vi "Generation of code word using msg and generator matrix(SubVI).vi"(1 "G in":dbl[][](array[numeric]), 2 "messages in":i16[][](array[numeric]), 3 "k":i32, 4 "n":i32) -> (0 "CODEWORDS":i32[][](array[numeric]))   [LabVIEW 2014]
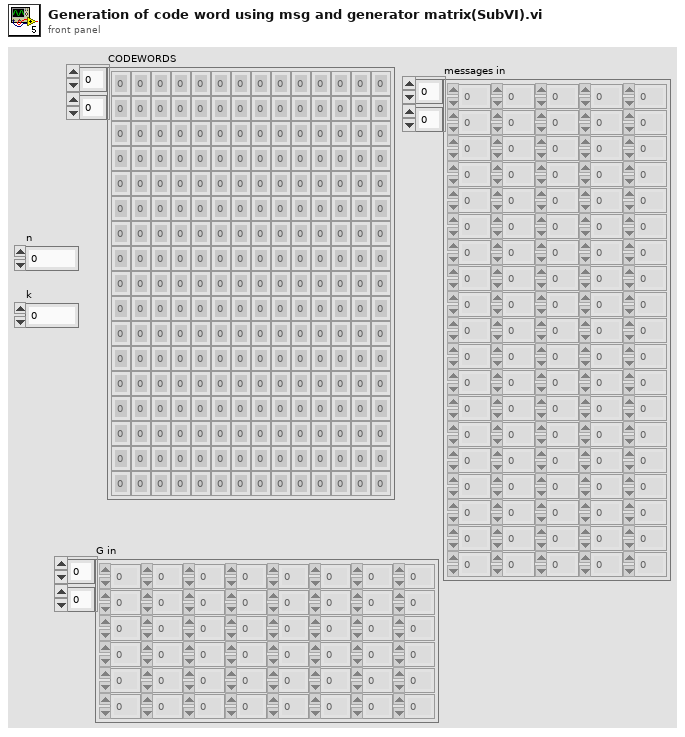
[diagram p1: front panel]
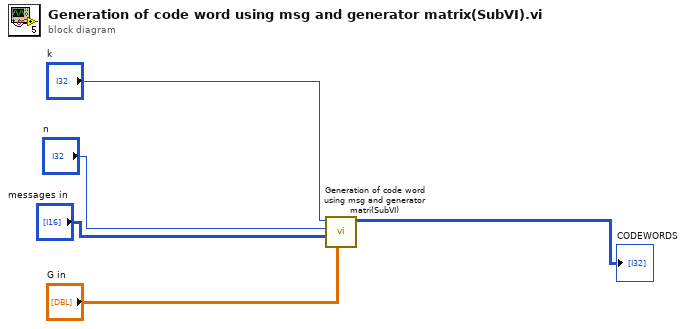
[diagram p0: block diagram]
diagram:
  n1 = call "Generation of code word using msg and generator matri(SubVI).vi"("G in"="G in", "messages in"="messages in", "n"="n", "k"="k") -> ("Array"=→"CODEWORDS":i32[][])  [unwired: 7 in]
